vi "variant_2d.vi"(3 "variant":variant) -> (1 "data":sgl[][](array[numeric]))   [LabVIEW 2014]
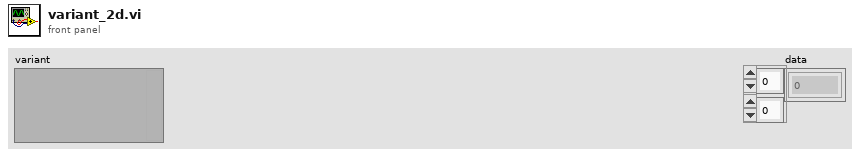
[diagram p1: front panel]
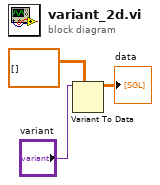
[diagram p0: block diagram]
diagram:
  n1 = Variant To Data(type=sgl[][] [], Variant="variant") -> (data=→"data":sgl[][])  [unwired: 1 in, 1 out]
